vi "CameraTest.vi"() -> ()   [LabVIEW 2016]
uses:
  <vilib>/userdefined/High Color/IMAQdx.ctl
  <vilib>/vision/driver/NI_Vision_Acquisition_Software.lvlib
panel:
  out "error out":errorcluster
  in  "stop":bool
  out "Image":T1(plugin-control)
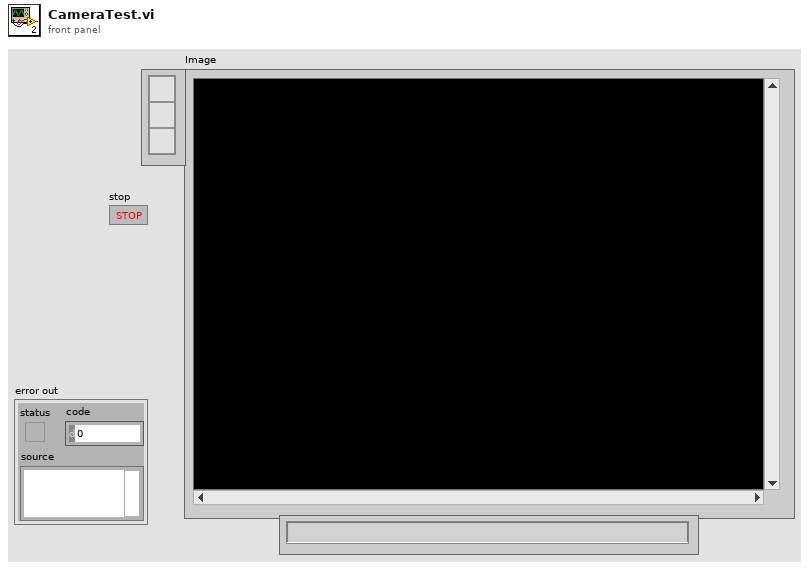
[diagram p1: front panel]
types:
  T1 = typedef "IMAQ Image.ctl" = refnum<image>
  T2 = typedef "IMAQdx.ctl" = refnum<k21>
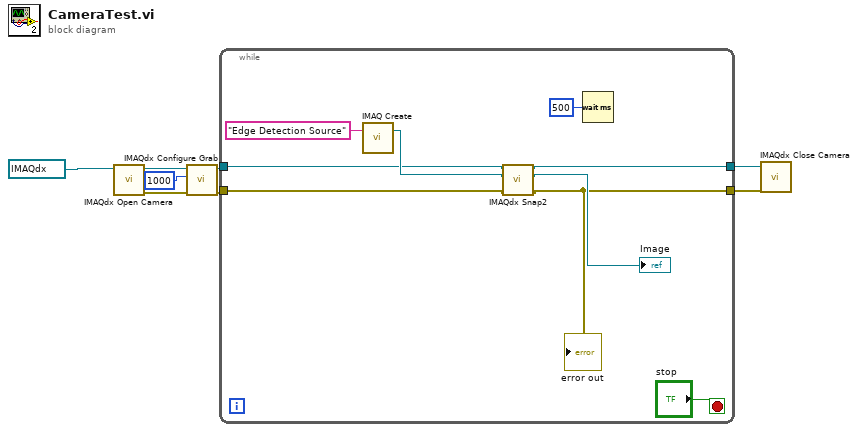
[diagram p0: block diagram]
diagram:
  n1 = call <vilib>:"IMAQdx Open Camera.vi"("Session In"=T2 "cam0") -> ("error out"=w7:errorcluster, "Session Out"=w8:T2)  [unwired: 9 in]
  n2 = call <vilib>:"IMAQdx Configure Grab.vi"("error in"=w7, "Number of Buffers"=u32 1000, "Session In"=w8) -> ("error out"=w5:errorcluster, "Session Out"=w6:T2)  [unwired: 7 in]
  n3 = while {
    tunnel: w6 -> [w12]
    tunnel: [w11] -> w3
    tunnel: w5 -> [w14]
    tunnel: [w9] -> w4
    stop <- "stop" stop-if-true
    n4 = call "IMAQ Create"("Image Name"="Edge Detection Source") -> ("New Image"=w13:T1)  [unwired: 4 in, 1 out]
    n5 = call <vilib>:"IMAQdx Snap2.vi"("error in"=w14, "Image In"=w13, "Session In"=w12) -> ("error out"=w9:errorcluster, "Image Out"=→"Image":T1, "Session Out"=w11:T2)  [unwired: 6 in]
    "error out" <- w9
    n6 = Wait (ms)(milliseconds to wait=u32 500) -> ()  [unwired: 1 out]
  }
  n7 = call <vilib>:"IMAQdx Close Camera.vi"("error in"=w4, "Session In"=w3) -> ()  [unwired: 9 in, 1 out]
